vi "Get Average Data from Array.vi"(8 "precision (6)":i16=3, 9 "Length":i32, 10 "Data":dbl, 11 "Array":dbl[](array[numeric])) -> (2 "mean":dbl format="%0.6f", 3 "Array Out":dbl[](array[numeric]))   [LabVIEW 2021]
uses:
  <vilib>/Analysis/NI_AALBase.lvlib
  <vilib>/Analysis/baseanly.llb/Mean (DBL).vi
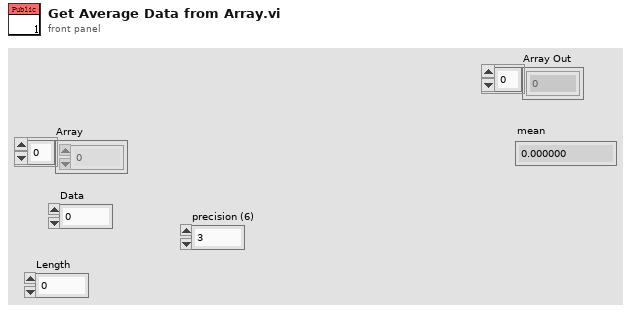
[diagram p1: front panel]
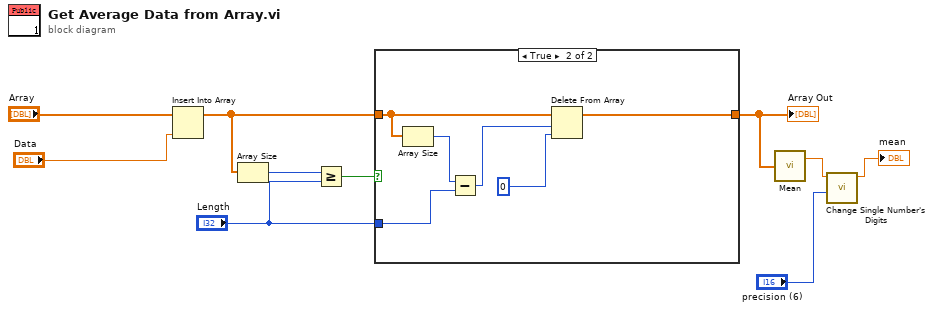
[diagram p0: block diagram]
diagram:
  n1 = Insert Into Array(array="Array", new element="Data") -> (w6:dbl[])  [unwired: 1 in]
  n2 = Array Size(array=w6) -> (size(s)=w8:i32)
  n3 = Greater Or Equal?(x=w8, y="Length") -> (x >= y?=w7:bool)
  n4 = case shown="True" w7 {
    tunnel: w6 -> [w11 w16]
    tunnel: [w11 w15] -> w4
    tunnel: "Length" -> [_ w13]
    frame False {
    }
    frame True {
      n5 = Array Size(array=w16) -> (size(s)=w14:i32)
      n6 = Subtract(x=w14, y=w13) -> (x-y=w12:i32)
      n7 = Delete From Array(array=w16, length=w12, index=0) -> (array with subset deleted=w15:dbl[])  [unwired: 1 out]
    }
  }
  "Array Out" <- w4
  n8 = call-poly <vilib>:"Mean.vi"("X"=w4) -> ("mean"=w3:dbl)  [unwired: 1 out]
  n9 = call <userlib>:"Change Single Number's Digits.vi"("precision (6)"="precision (6)", "number"=w3) -> ("number 2"=→"mean":dbl)  [unwired: 8 in, 1 out]
